vi "Process.vi"(8 "error in":errorcluster, 11 "Oxford1820 UI in":refnum<class "Instrument.OxfordVRM UI.lvclass">) -> (0 "error out":errorcluster, 3 "Oxford1820 UI out":refnum<class "Instrument.OxfordVRM UI.lvclass">)   [LabVIEW 2016, in "Instrument.OxfordVRM UI.lvclass"]
doc: "---------------------------------------------------------------\nJKI State Machine Objects™\nhttp://jki.net/state-machine-objects/\nCopyright (C) 2005-2015, JKI <info@jki.net>\nALL RIGHTS RESERVEDJKI State Machine Objects (SMO) 1.0.0.5\nJKI - JKI\nCopyright (c) 2016, JKI"
uses:
  Instrument.OxfordVRM UI.lvclass
  <vilib>/JKI/JKI SMO/SMO/SMO.lvclass
  <vilib>/JKI/JKI SMO/SMO/Typedefs/Parent Call--Enum.ctl
  <vilib>/JKI/JKI SMO/SMO.UI/SMO.UI.lvclass
  <userlib>/LevyLab/Levylab Instruments/SMOs/Instrument/Instrument.lvclass
  Instrument.Oxford1820/Typedefs/getAll.ctl
  Instrument.Oxford1820/Instrument.OxfordVRM.lvclass
  <userlib>/LevyLab/Levylab Instruments/SMOs/Instrument UI/Instrument UI.lvclass
  Instrument.Oxford1820/Typedefs/Fill Mode-Combo.ctl
  <instrlib>/Mercury iXX/Public/Libraries/Magnet/Controls/Switch Heater.ctl
  <instrlib>/Mercury iXX/Public/Libraries/Magnet.lvlib
  C:/Program Files (x86)/National Instruments/LabVIEW 2016/user.lib/LevyLab/Levylab Instruments/SMOs/Instrument UI/Instrument UI.lvclass
  C:/Program Files (x86)/National Instruments/LabVIEW 2016/vi.lib/JKI/JKI SMO/SMO.UI/SMO.UI.lvclass
  C:/Program Files (x86)/National Instruments/LabVIEW 2016/vi.lib/JKI/JKI SMO/SMO/SMO.lvclass
  C:/Program Files (x86)/National Instruments/LabVIEW 2016/user.lib/LevyLab/Levylab Instruments/Instrument Types/Cryostat/Instrument.Cryostat.lvclass
  C:/Program Files (x86)/National Instruments/LabVIEW 2016/user.lib/LevyLab/Levylab Instruments/SMOs/Instrument/Instrument.lvclass
panel:
  in  "Open Target":dbl=100.0 format="%.1f (%%)"
  out "System Time (HH:MM:SS)":dbl=165.3592643737793 format="%<%I:%M:%S %p>T"
  out "LPF on":dbl format="%<%H:%M:%S>t"
  out "PS Heat on (HH:MM:SS)":dbl format="%<%H:%M:%S>t"
  out "ETA":dbl=3660699600.0 format="%<%I:%M:%S %p %m/%d/%Y>T"
  out "version":string="v20/10/28"
  out "Waveform Chart 2":T1(graph)
  out "N2 LEVEL":dbl format="%.0f %"
  in  "Window Maximize":bool
  in  "Window Minimize":bool
  out "Magnet Status 3":string="Status: Clamped"
  in  "Remote Mode":bool
  out "Sentinel":bool=TRUE
  out "Voltage Meter":dbl(knob) caption="Voltage (V)" scale=-10.0..10.0
  out "Current Meter":dbl(knob) caption="Voltage (V)" scale=-180.0..180.0
  out "Magnet Field Meter":dbl(knob) caption="Voltage (V)" scale=-20.0..20.0
  in  "Hold":bool
  in  "To Set":bool
  in  "Export":bool
  out "PSU Field":dbl format="%#.5f T"
  in  "Target Field (T)":dbl caption="Field" format="%.2f"
  out "Target Field (T)":dbl caption="Field" format="%.2f T"
  in  "Target Rate (T/min)":dbl=0.1 caption="Rate" min=0.0 max=1.0 format="%.2f"
  out "Target Rate (T/min)":dbl caption="Rate" format="%.2f T/min"
  out "Field":dbl format="%.5f T"
  out "He LEVEL":dbl format="%.0f %"
  in  "PS Heat":bool
  in  "To Zero":bool
  in  "Clamp":bool
  out "N2 LVL":dbl format="%.1f (%%)"
  out "He LVL Chart":dbl(slide)=52.0833 scale=0.0..100.0
  out "N2 LVL Chart":dbl(slide)=61.3025 scale=0.0..100.0
  out "He LVL":dbl format="%.1f (%%)"
  in  "Fast/Slow Fill":bool
  in  "Open Needle Valve":bool
  in  "Close Needle Valve":bool
  in  "LPF Power":bool
  out "Needle Valve":dbl format="%.1f (%%)"
  out "Pressure":dbl format="%_5f mB"
  out "Magnet T":dbl format="%_2f K"
  out "Magnet R":dbl format="%_3f ohms"
  out "Voltage":dbl format="%.5f V"
  out "Current":dbl format="%.5f A"
  out "Magnet Status 2":string="Status: Clamped"
  in  "Power":bool
  # "Obsolete controls?"
  # "Actions"
  # "Targets"
  # "Status"
  # "Slow Rates\nCurrent Range (A)     Field Range (T)  Rate (T/min)\n0       -- 100        0    -- 11.5     0.91\n100     -- 150        11.5 -- 17.2     0.23\n150     -- 155.467    17.2 -- 18       0.11\n155.567 -- 172.471    18   -- 20       0.11\n\nFast Rates\nCurrent Range (A)     Field Range (T)  Rate (T/min)\n0       -- 155.467    0    -- 18       1.0\n155.567 -- 172.471    18   -- 20       0.25"
  # "IPS"
  # "PS Switch"
  # "Level"
  # "Level Graph"
  # "LPF"
  # "Helium"
  # "Nitrogen"
  # "^^^^"
  # "Needle Valve"
  # "Slow Rates\nCurrent Range (A)     Field Range (T)   Rate (T/min)\n0       -- 100        0    -- 11.5      0.91\n100     -- 150        11.5 -- 17.2      0.23\n150     -- 155.467    17.2 -- 18        0.11\n155.567 -- 172.471    18   -- 20        0.11\n\nFast Rates\nCurrent Range (A)     Field Range (T)   Rate (T/min)\n0       -- 155.467    0    -- 18        1.0\n155.567 -- 172.471    18   -- 20        0.25"
  # "SMO UI Template"
  # "For instructions on how to use the JKI State Machine Objects, examples and video tutorials, visit:\nhttp://jki.net/state-machine-objects/\n\nJKI State Machine Objects™\nhttp://jki.net/state-machine-objects/\nCopyright (C) 2005-2015, JKI <info@jki.net>\nALL RIGHTS RESERVED"
  # "Voltage (V)"
  # "Current (A)"
  # "Magnet (T)"
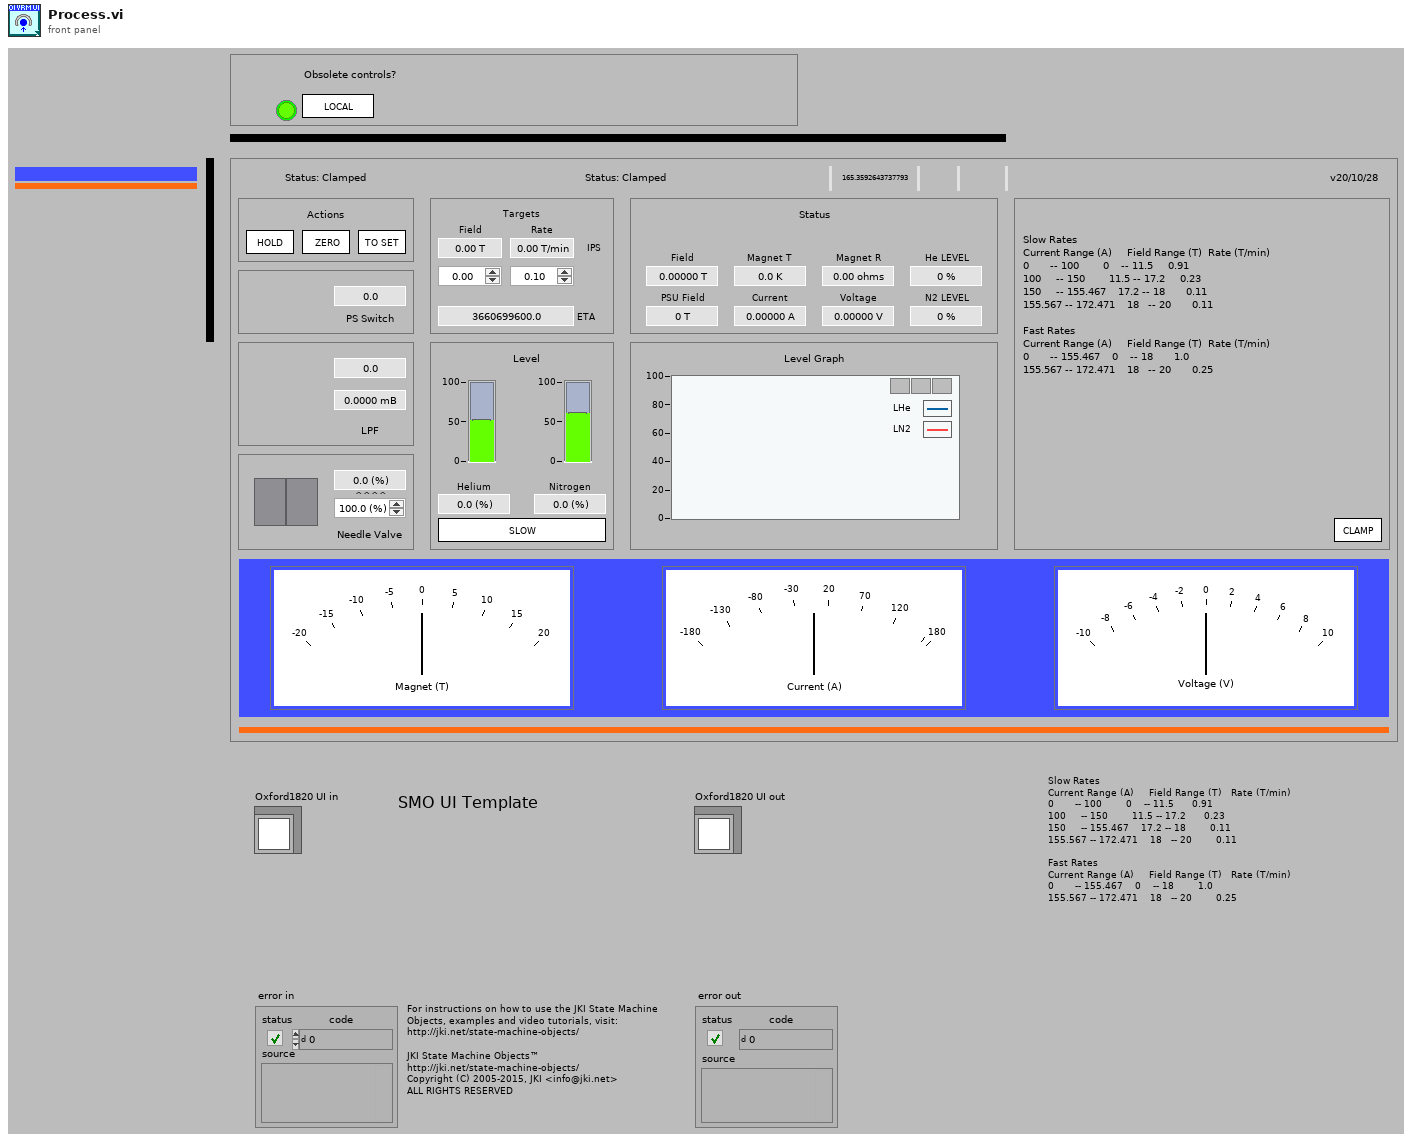
[diagram p1: front panel]
types:
  T1 = cluster{"1820_IPS_Level_He":dbl, "1820_IPS_Level_N2":dbl}
  T2 = typedef "SMO.lvclass/Parent Call--Enum.ctl" = enum16{"Allows parent to run", "Does not request parent to run"}
  T3 = typedef "Mercury iXX.lvlib/Magnet.lvlib/Switch Heater.ctl" = string
  T4 = enum32{"invalid app kind", "Development System", "Run Time System", "Student Edition", "Embedded LabVIEW", "Evaluation", "Custom"}
  T5 = typedef "Instrument.OxfordVRM.lvclass/getAll.ctl" = cluster{"1820_IPS_Magnet_Field":dbl, "1820_IPS_PS_Field":dbl, "1820_IPS_Target_Field":dbl, "1820_IPS_Target_Field_Rate":dbl, "1820_IPS_Voltage":dbl, "1820_IPS_Current":dbl, "1820_IPS_Level_N2":dbl, "1820_IPS_Level_He":dbl, "1820_IPS_Magnet_Temperature":dbl, "1820_IPS_Magnet_Temperature_R":dbl, "1820_IPS_M1_Current":dbl, "1820_IPS_M1_Voltage":dbl, "1820_IPS_M2_Current":dbl, "1820_IPS_M2_Voltage":dbl, "1820_IPS_M3_Current":dbl, "1820_IPS_M3_Voltage":dbl, "1820_IPS_Status":string, "1820_IPS_Switch":string, "1820_ITC_Lambda_Temperature":dbl, "1820_ITC_Lambda_Temperature_R":dbl, "1820_ITC_Pressure":dbl, "1820_ITC_Needle_Valve":dbl}
  T6 = enum32{"Invalid", "Standard", "Closed", "Hidden", "Minimized", "Maximized"}
  T7 = typedef "Instrument.OxfordVRM.lvclass/Fill Mode-Combo.ctl" = string
  T8 = typedef "RemoteControl.lvclass/Message--Cluster.ctl" = cluster{"Command":string, "Data":variant, "Message ID":i32}
  T9 = cluster{"Core":cluster{"Current VI Reference":refnum<vi>, "Close Panel on Exit?":bool, "error":errorcluster}, "Instrument UI out":refnum<class "Instrument.OxfordVRM UI.lvclass">, "Instrument":refnum<class "Instrument.OxfordVRM.lvclass">, "getAll":variant, "Response":string, "config":variant, "switch time":timestamp, "LPF time":timestamp}
  T10 = typedef "Instrument.OxfordVRM.lvclass/PublicEvents--Instrument.Oxford1820.ProcessStatus.ctl" = string
  T11 = cluster{"Current VI Reference":refnum<vi>, "Close Panel on Exit?":bool, "error":errorcluster}
  T12 = typedef "LVRectTypeDef.ctl" = cluster{"Left":i16, "Top":i16, "Right":i16, "Bottom":i16}
  T13 = typedef "SMO.lvclass/Protected Events.ctl" = cluster{"StopProcesses":refnum<user-event>, "AbortProcesses":refnum<user-event>, "Config Changed":refnum<user-event>, "Dependency":refnum<user-event>}
  T14 = typedef "Instrument.lvclass/PublicEvents--Cluster.ctl" = cluster{"MessageFromProcess":refnum<user-event>}
  T15 = typedef "Instrument.OxfordVRM.lvclass/PublicEvents--Cluster.ctl" = cluster{"ProcessStatus":refnum<user-event>}
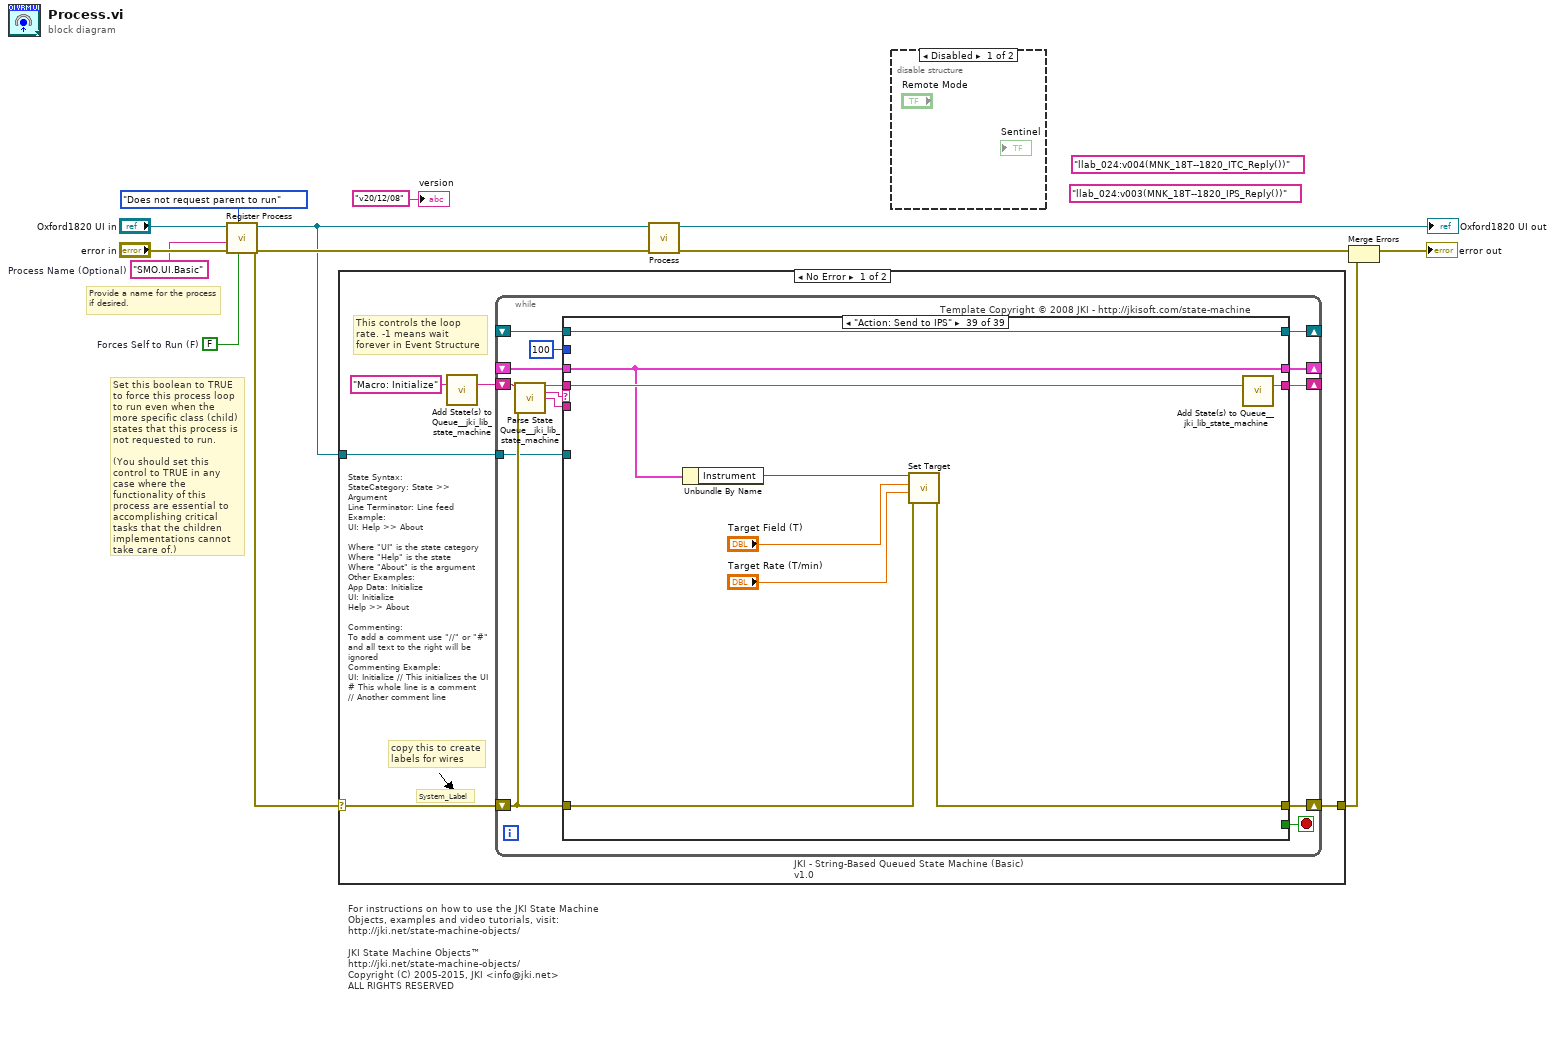
[diagram p0: block diagram]
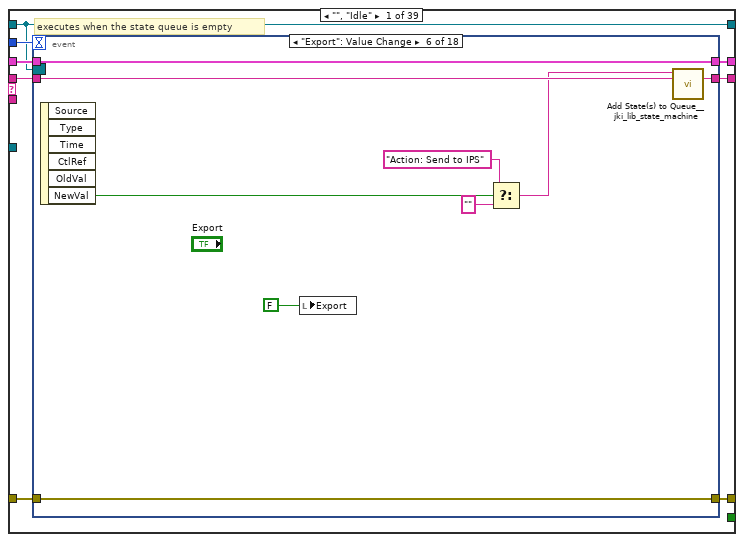
[diagram p3: hidden frame]
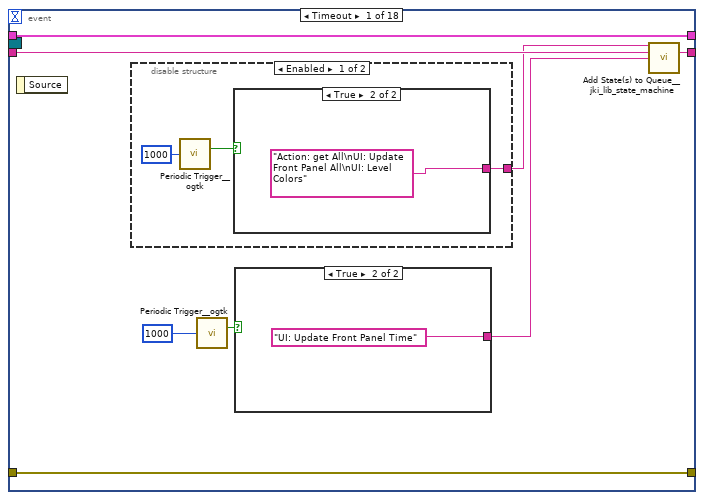
[diagram p4: hidden frame]
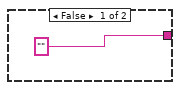
[diagram p5: hidden frame]
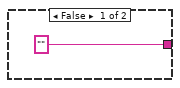
[diagram p6: hidden frame]
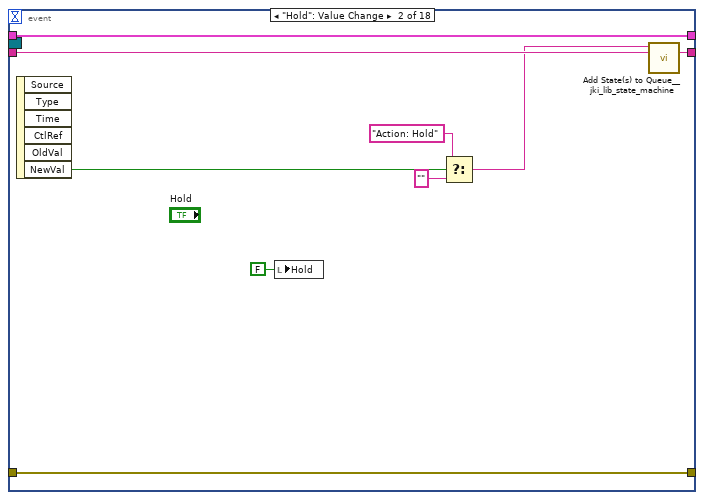
[diagram p8: hidden frame]
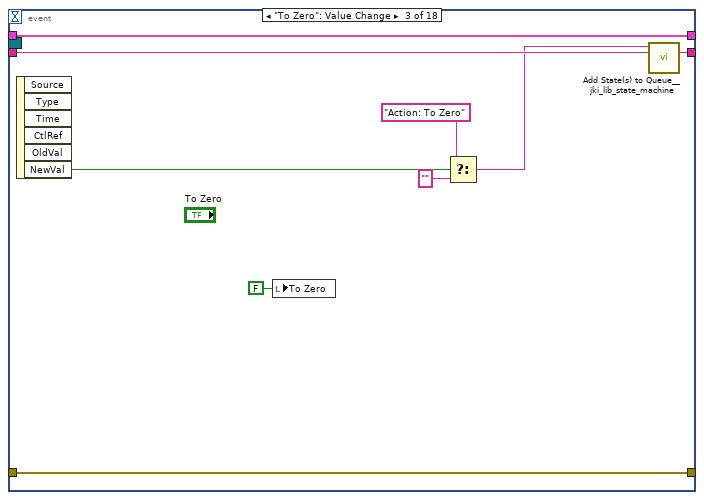
[diagram p9: hidden frame]
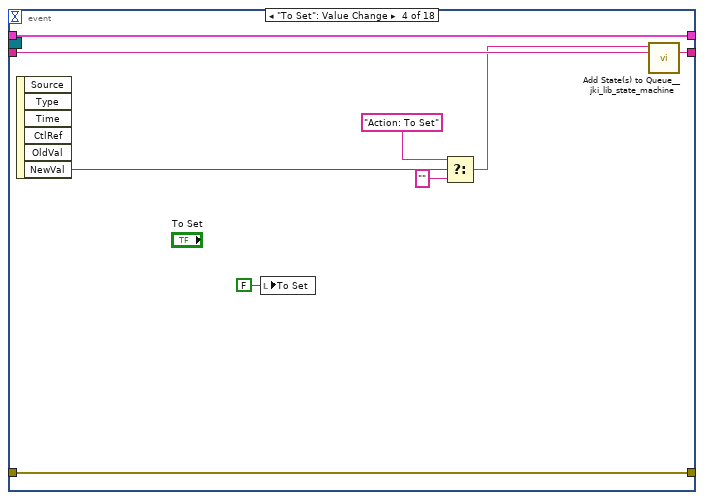
[diagram p10: hidden frame]
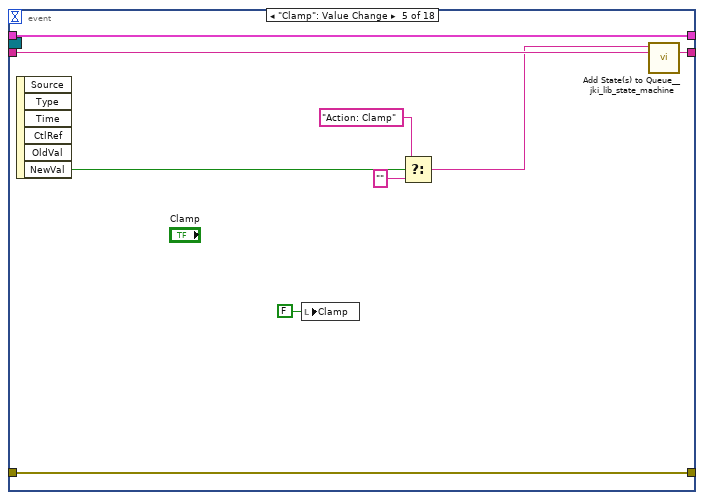
[diagram p11: hidden frame]
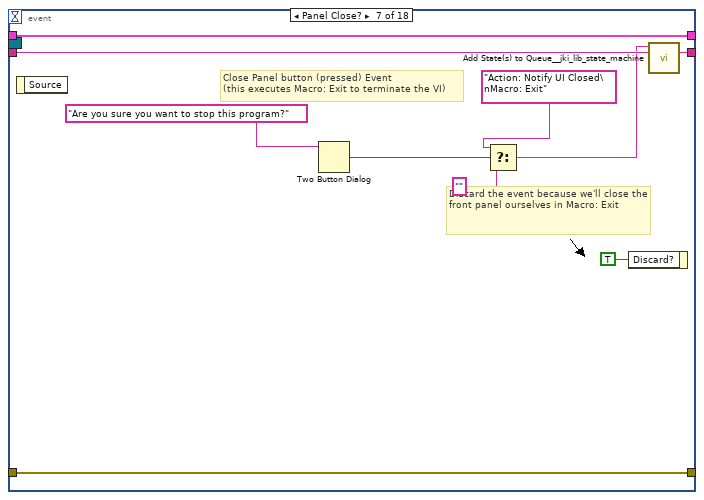
[diagram p12: hidden frame]
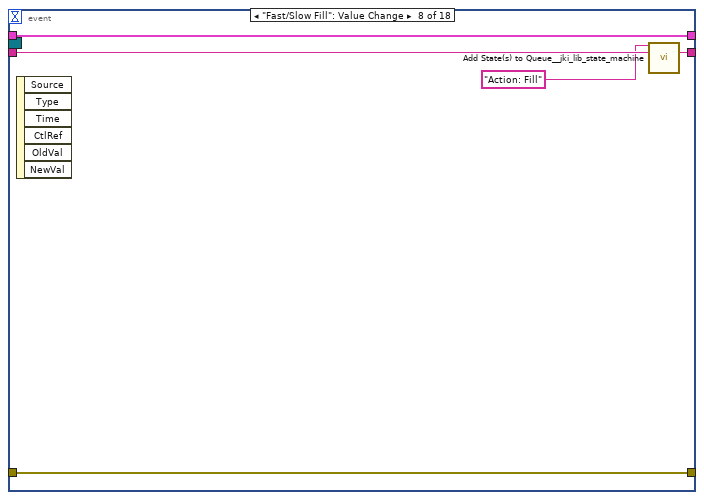
[diagram p13: hidden frame]
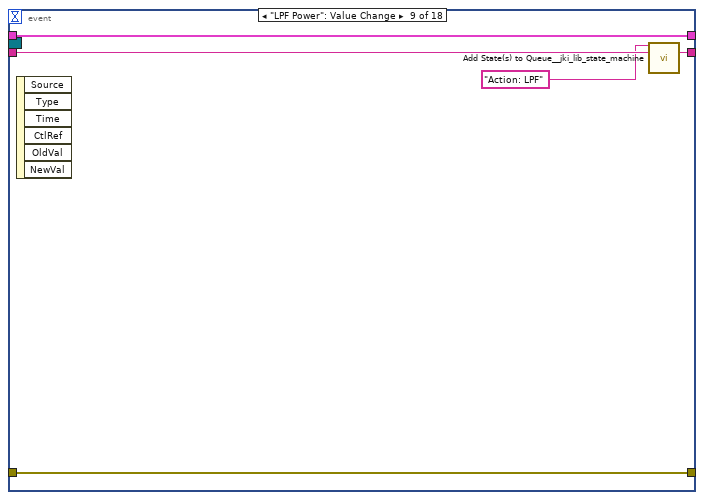
[diagram p14: hidden frame]
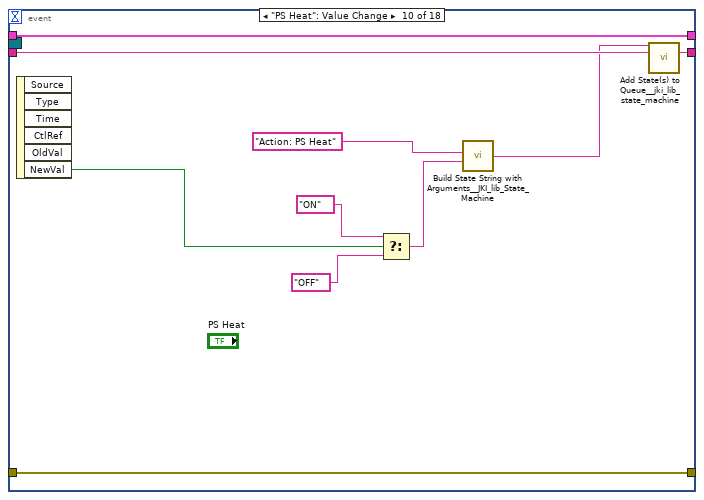
[diagram p15: hidden frame]
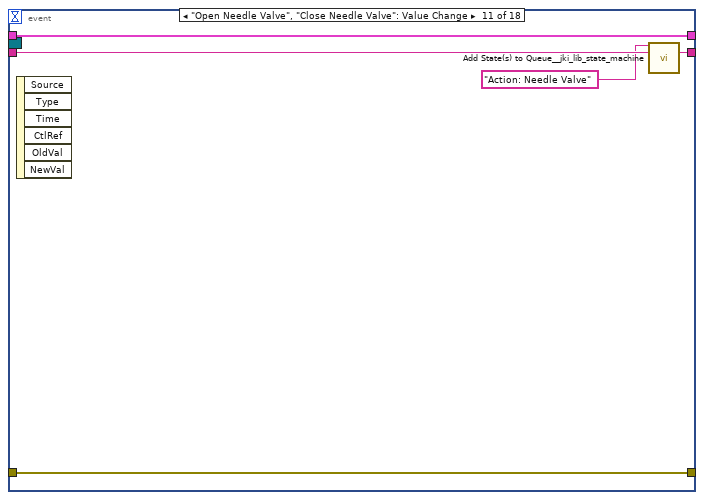
[diagram p16: hidden frame]
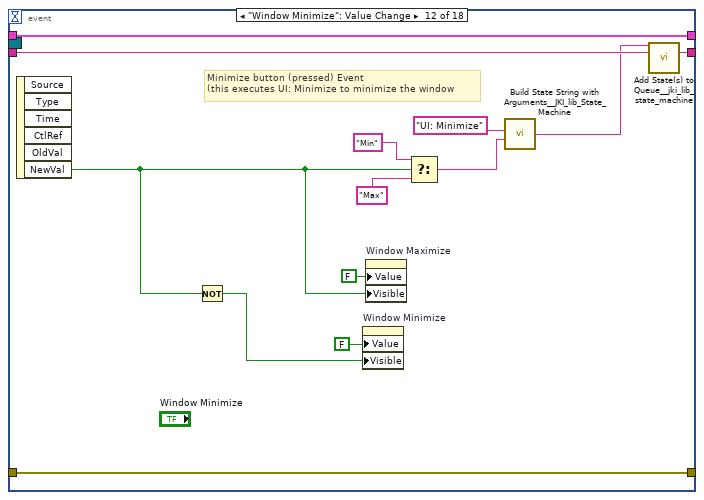
[diagram p17: hidden frame]
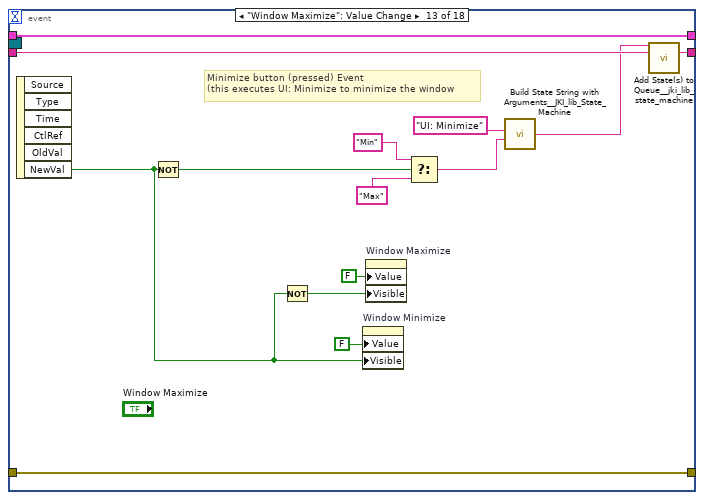
[diagram p18: hidden frame]
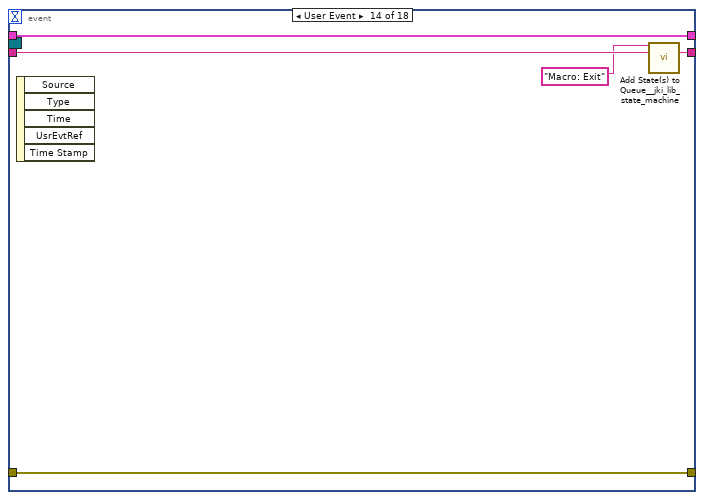
[diagram p19: hidden frame]
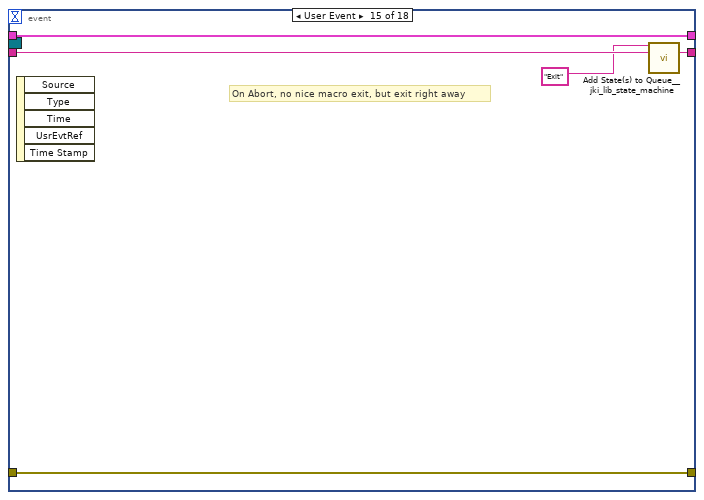
[diagram p20: hidden frame]
diagram:
  (unwired) "llab_024:v004(MNK_18T--1820_ITC_Reply())" ("variable")
  (unwired) "llab_024:v003(MNK_18T--1820_IPS_Reply())" ("variable")
  w3 = FALSE  # Forces Self to Run (F)
  w2 = "SMO.UI.Basic"  # Process Name (Optional)
  # "Provide a name for the process\nif desired."
  # "Set this boolean to TRUE to force this process loop to run even when the more specific class (child) states that this process is not requested to run.\n\n(You should set this control to TRUE in any case where the functionality of this process are essential to accomplishing critical tasks that the children implementations cannot take care of.)"
  # "For instructions on how to use the JKI State Machine Objects, examples and video tutorials, visit:\nhttp://jki.net/state-machine-objects/\n\nJKI State Machine Objects™\nhttp://jki.net/state-machine-objects/\nCopyright (C) 2005-2015, JKI <info@jki.net>\nALL RIGHTS RESERVED"
  n1 = call <vilib>:"Register Process.vi"("Forces Self to Run (F)"=w3, "Parent Call"=Parent_Call--Enum."Does not request parent to run", "error in (no error)"="error in", "Process Name (optional)"=w2, "SMO"="Oxford1820 UI in") -> ("error out"=w9:errorcluster, "SMO out"=w8:refnum<class "Instrument.OxfordVRM UI.lvclass">)  [unwired: 5 in]
  n2 = case shown="No Error" w9 {
    selector: w9 -> [w14 w643]
    tunnel: w8 -> [w15 _]
    tunnel: [w13 w643] -> w5
    frame No Error {
      # "State Syntax:\nStateCategory: State >> Argument\nLine Terminator: Line feed\nExample:\nUI: Help >> About\n\nWhere \"UI\" is the state category\nWhere \"Help\" is the state\nWhere \"About\" is the argument\nOther Examples:\nApp Data: Initialize\nUI: Initialize\nHelp >> About\n\nCommenting:\nTo add a comment use \"//\" or \"#\" and all text to the right will be ignored\nCommenting Example:\nUI: Initialize // This initializes the UI\n# This whole line is a comment\n// Another comment line"
      # "copy this to create labels for wires"
      # "This controls the loop rate. -1 means wait forever in Event Structure"
      # "System_Label"
      n3 = call <vilib>:"Add State(s) to Queue__jki_lib_state_machine.vi"("State(s) in (\"\")"="Macro: Initialize") -> ("States Out"=w17:string)  [unwired: 14 in]
      n4 = while "JKI - String-Based Queued State Machine (Basic) v1.0" {
        shift-right: [w24] -> _
        shift-left: _ -> [w23]
        shift-right: [w27] -> w13
        shift-left: w14 -> [w21]
        shift-right: [w26] -> _
        shift-left: w17 -> [w28]
        tunnel: w15 -> [w20]
        shift-right: [w19] -> _
        shift-left: _ -> [w18]
        stop <- w25 stop-if-true
        # "Template Copyright © 2008 JKI - http://jkisoft.com/state-machine"
        n5 = call <vilib>:"Parse State Queue__jki_lib_state_machine.vi"("State Queue"=w28, "Error In (no error)"=w21) -> ("Remaining States"=w30:string, "Current State"=w31:string, "Arguments"=w29:string)  [unwired: 11 in]
        n6 = case shown="\"Action: Send to IPS\"" w31 {
          selector: w31 -> [_ _ w219 _ _ _ _ _ _ _ _ _ _ _ _ _ _ _ _ _ _ _ _ _ _ _ _ _ _ _ _ _ _ _ _ _ _ _ _]
          tunnel: w30 -> [w39 w217 w223 w242 w256 w262 w267 w290 w297 w302 w313 w339 w358 w364 w371 w378 w394 w428 w454 w463 w477 w482 w493 w500 w505 w521 w527 w534 w541 w551 w560 w567 w574 w581 w592 w605 w618 w633 w642]
          tunnel: w29 -> [_ _ _ _ _ _ _ _ _ _ _ _ _ w359 _ w372 w388 w429 _ _ _ _ _ _ _ _ _ _ _ _ _ _ _ _ _ _ _ w624 _]
          tunnel: w23 -> [w37 w214 w221 w233 w244 w258 w264 _ w292 w299 w311 w336 w354 w361 w368 w376 w390 w427 w451 w459 w468 w479 w490 w495 w502 w519 w525 w530 w537 w542 w557 w564 w571 w575 w589 w595 w615 w628 w639]
          tunnel: [w36 w215 w225 w239 w249 w257 w265 w278 w293 w300 w308 w334 w356 w362 w369 w373 w391 w422 w452 w461 w475 w480 w484 w496 w503 w515 w522 w531 w535 w545 w556 w561 w568 w576 w586 w600 w606 w629 w636] -> w27
          tunnel: w21 -> [w35 w215 w224 w239 w245 _ w265 w287 w294 w300 w309 w335 w356 w362 w369 w374 w392 w423 w452 w461 w475 w480 w485 w497 w503 w510 w523 w531 w536 w546 w553 w562 w569 w577 w587 w601 w613 w630 w637]
          tunnel: [w38 w216 w222 w241 w255 w261 w266 w289 w296 w301 w312 w338 w357 w363 w370 w377 w393 w433 w453 w462 w476 w481 w492 w499 w504 w520 w526 w533 w540 w550 w559 w566 w573 w580 w591 w604 w617 w632 w641] -> w26
          tunnel: [_ _ _ _ _ TRUE _ _ _ _ _ _ _ _ _ _ _ _ _ _ _ _ _ _ _ _ _ _ _ _ _ _ _ _ _ _ _ _ _] -> w25
          tunnel: [w34 w214 w221 w240 w247 w258 w264 w288 w292 w299 w311 w336 w354 w361 w368 w376 w390 w427 w451 w459 w468 w479 w490 w495 w502 w519 w525 w529 w537 w548 w557 w564 w571 w575 w589 w594 w615 w626 w639] -> w24
          tunnel: 100 ("Timeout") -> [w33 _ _ _ _ _ _ _ _ _ _ _ _ _ _ _ _ _ _ _ _ _ _ _ _ _ _ _ _ _ _ _ _ _ _ _ _ _ _]
          tunnel: w20 -> [_ _ _ _ _ _ _ w275 _ _ _ _ _ _ _ _ _ _ _ _ _ _ _ _ _ _ _ _ _ _ _ _ _ _ _ _ _ _ _]
          tunnel: [w32 w213 w218 w230 w254 w259 w263 w285 w291 w298 w310 w337 w355 w360 w367 w375 w387 w432 w450 w460 w469 w478 w491 w498 w501 w518 w524 w532 w539 w549 w558 w565 w572 w579 w590 w603 w616 w631 w640] -> w19
          tunnel: w18 -> [w32 w213 w218 w230 w254 w259 w263 w285 w291 w298 w310 w337 w355 w360 w367 w375 w387 w432 w450 w460 w469 w478 w491 w498 w501 _ w524 w532 w539 w549 w558 w565 w572 w579 w590 w603 w616 w631 w640]
          frame "", "Idle" {
            # "executes when the state queue is empty"
            n7 = event shown="[5] \"Export\": Value Change" {
              selector: w32 -> [_ _ _ _ _ _ _ _ _ _ _ _ _ _ _ _ _ _]
              dyn-events: _ -> [_ _ _ _ _ _ _ _ _ _ _ _ _ _ _ _ _ _]
              timeout: w33 -> [_ _ _ _ _ _ _ _ _ _ _ _ _ _ _ _ _ _]
              tunnel: w39 -> [w47 w63 w72 w81 w90 w99 w109 w114 w119 w129 w134 w147 w161 w166 w171 w180 w190 w212]
              tunnel: [w46 w62 w71 w80 w89 w98 w108 w113 w118 w128 w133 w146 w160 w165 w170 w179 w189 w211] -> w38
              tunnel: w37 -> [w43 w60 w69 w78 w87 w96 w106 w112 w117 w127 w132 w145 w159 w163 w168 w177 w188 w205]
              tunnel: [w45 w61 w70 w79 w88 w97 w105 w111 w116 w126 w131 w144 w158 w164 w169 w178 w181 w209] -> w36
              tunnel: w35 -> [w45 w61 w70 w79 w88 w97 w105 w111 w116 w126 w131 w144 w158 w164 w169 w178 w182 w206]
              tunnel: [w43 w60 w69 w78 w87 w96 w106 w112 w117 w127 w132 w145 w159 w163 w168 w177 w187 w205] -> w34
              event Timeout {
                n8 = event-data() -> ()  [unwired: 1 in, 1 out]
                n9 = disable-structure shown="Enabled" {
                  disable-tunnel: [w50 _] -> w44
                  frame Enabled {
                    n10 = call <userlib>:"Periodic Trigger__ogtk.vi"("time (ms)"=u32 1000 ("update time (ms)")) -> ("Triggered"=w52:bool)  [unwired: 12 in, 2 out]
                    n11 = case shown="True" w52 {
                      tunnel: ["" "Action: get All\nUI: Update Front Panel All\nUI: Level Colors"] -> w50
                      frame False {
                      }
                      frame True {
                      }
                    }
                  }
                  frame Disabled {
                  }
                }
                n12 = call <userlib>:"Periodic Trigger__ogtk.vi"("time (ms)"=u32 1000 ("update time (ms)")) -> ("Triggered"=w41:bool)  [unwired: 12 in, 2 out]
                n13 = case shown="True" w41 {
                  tunnel: ["" "UI: Update Front Panel Time"] -> w40
                  frame False {
                  }
                  frame True {
                  }
                }
                n14 = call <vilib>:"Add State(s) to Queue__jki_lib_state_machine.vi"("State(s) in Front (\"\")"=w44, "State(s) in (\"\")"=w47, "State(s) at Back (\"\")"=w40) -> ("States Out"=w46:string)  [unwired: 12 in]
              }
              event "Hold": Value Change {
                n15 = event-data() -> ("NewVal"=w59:bool)  [unwired: 1 in, 5 out]
                n16 = local write "Hold"(FALSE ("Hold")) -> ()
                n17 = Select(t="Action: Hold" ("State(s) in Front (\"\")"), s=w59, f="") -> (s? t:f=w56:string)
                n18 = call <vilib>:"Add State(s) to Queue__jki_lib_state_machine.vi"("State(s) in Front (\"\")"=w56, "State(s) in (\"\")"=w63) -> ("States Out"=w62:string)  [unwired: 13 in]
              }
              event "To Zero": Value Change {
                n19 = event-data() -> ("NewVal"=w67:bool)  [unwired: 1 in, 5 out]
                n20 = local write "To Zero"(FALSE ("To Zero")) -> ()
                n21 = Select(t="Action: To Zero" ("State(s) in Front (\"\")"), s=w67, f="") -> (s? t:f=w65:string)
                n22 = call <vilib>:"Add State(s) to Queue__jki_lib_state_machine.vi"("State(s) in Front (\"\")"=w65, "State(s) in (\"\")"=w72) -> ("States Out"=w71:string)  [unwired: 13 in]
              }
              event "To Set": Value Change {
                n23 = event-data() -> ("NewVal"=w76:bool)  [unwired: 1 in, 5 out]
                n24 = local write "To Set"(FALSE ("To Set")) -> ()
                n25 = Select(t="Action: To Set" ("State(s) in Front (\"\")"), s=w76, f="") -> (s? t:f=w74:string)
                n26 = call <vilib>:"Add State(s) to Queue__jki_lib_state_machine.vi"("State(s) in Front (\"\")"=w74, "State(s) in (\"\")"=w81) -> ("States Out"=w80:string)  [unwired: 13 in]
              }
              event "Clamp": Value Change {
                n27 = event-data() -> ("NewVal"=w85:bool)  [unwired: 1 in, 5 out]
                n28 = local write "Clamp"(FALSE ("Clamp")) -> ()
                n29 = Select(t="Action: Clamp" ("State(s) in Front (\"\")"), s=w85, f="") -> (s? t:f=w83:string)
                n30 = call <vilib>:"Add State(s) to Queue__jki_lib_state_machine.vi"("State(s) in Front (\"\")"=w83, "State(s) in (\"\")"=w90) -> ("States Out"=w89:string)  [unwired: 13 in]
              }
              event "Export": Value Change {
                n31 = event-data() -> ("NewVal"=w95:bool)  [unwired: 1 in, 5 out]
                n32 = local write "Export"(FALSE ("Send to IPS")) -> ()
                n33 = Select(t="Action: Send to IPS" ("State(s) in Front (\"\")"), s=w95, f="") -> (s? t:f=w92:string)
                n34 = call <vilib>:"Add State(s) to Queue__jki_lib_state_machine.vi"("State(s) in Front (\"\")"=w92, "State(s) in (\"\")"=w99) -> ("States Out"=w98:string)  [unwired: 13 in]
              }
              event Panel Close? {
                # "Discard the event because we'll close the front panel ourselves in Macro: Exit"
                # "Close Panel button (pressed) Event\n(this executes Macro: Exit to terminate the VI)"
                n35 = event-data() -> ()  [unwired: 1 in, 1 out]
                n36 = Two Button Dialog(message="Are you sure you want to stop this program?") -> (T button?=w104:bool)  [unwired: 2 in]
                n37 = Select(t="Action: Notify UI Closed\nMacro: Exit", s=w104, f="") -> (s? t:f=w100:string)
                n38 = event-data("Discard?"=TRUE) -> ()  [unwired: 1 in, 1 out]
                n39 = call <vilib>:"Add State(s) to Queue__jki_lib_state_machine.vi"("State(s) in Front (\"\")"=w100, "State(s) in (\"\")"=w109) -> ("States Out"=w108:string)  [unwired: 13 in]
              }
              event "Fast/Slow Fill": Value Change {
                n40 = event-data() -> ()  [unwired: 1 in, 6 out]
                n41 = call <vilib>:"Add State(s) to Queue__jki_lib_state_machine.vi"("State(s) in Front (\"\")"="Action: Fill", "State(s) in (\"\")"=w114) -> ("States Out"=w113:string)  [unwired: 13 in]
              }
              event "LPF Power": Value Change {
                n42 = event-data() -> ()  [unwired: 1 in, 6 out]
                n43 = call <vilib>:"Add State(s) to Queue__jki_lib_state_machine.vi"("State(s) in Front (\"\")"="Action: LPF", "State(s) in (\"\")"=w119) -> ("States Out"=w118:string)  [unwired: 13 in]
              }
              event "PS Heat": Value Change {
                n44 = event-data() -> ("NewVal"=w120:bool)  [unwired: 1 in, 5 out]
                n45 = Select(t=T3 "ON" ("LPF State"), s=w120, f=T3 "OFF" ("LPF State")) -> (s? t:f=w122:T3)
                n46 = call <vilib>:"Build State String with Arguments__JKI_lib_State_Machine.vi"("Arguments (\"\")"=w122, "State"="Action: PS Heat") -> ("State with Arguments"=w121:string)  [unwired: 4 in]
                n47 = call <vilib>:"Add State(s) to Queue__jki_lib_state_machine.vi"("State(s) in Front (\"\")"=w121, "State(s) in (\"\")"=w129) -> ("States Out"=w128:string)  [unwired: 13 in]
              }
              event "Open Needle Valve", "Close Needle Valve": Value Change {
                n48 = event-data() -> ()  [unwired: 1 in, 6 out]
                n49 = call <vilib>:"Add State(s) to Queue__jki_lib_state_machine.vi"("State(s) in Front (\"\")"="Action: Needle Valve", "State(s) in (\"\")"=w134) -> ("States Out"=w133:string)  [unwired: 13 in]
              }
              event "Window Minimize": Value Change {
                # "Minimize button (pressed) Event\n(this executes UI: Minimize to minimize the window"
                n50 = event-data() -> ("NewVal"=w135:bool)  [unwired: 1 in, 5 out]
                n51 = Not(x=w135) -> (.not. x?=w136:bool)
                n52 = property on="Window Minimize" class="Bool (strict)"("Value"=FALSE ("Window Maximize"), "Visible"=w136) -> ()  [unwired: 2 in, 2 out]
                n53 = property on="Window Maximize" class="Bool (strict)"("Value"=FALSE ("Window Maximize"), "Visible"=w135) -> ()  [unwired: 2 in, 2 out]
                n54 = Select(t="Min" ("Arguments (\"\")"), s=w135, f="Max" ("Arguments (\"\")")) -> (s? t:f=w140:string)
                n55 = call <vilib>:"Build State String with Arguments__JKI_lib_State_Machine.vi"("Arguments (\"\")"=w140, "State"="UI: Minimize") -> ("State with Arguments"=w139:string)  [unwired: 4 in]
                n56 = call <vilib>:"Add State(s) to Queue__jki_lib_state_machine.vi"("State(s) in Front (\"\")"=w139, "State(s) in (\"\")"=w147) -> ("States Out"=w146:string)  [unwired: 13 in]
              }
              event "Window Maximize": Value Change {
                # "Minimize button (pressed) Event\n(this executes UI: Minimize to minimize the window"
                n57 = event-data() -> ("NewVal"=w149:bool)  [unwired: 1 in, 5 out]
                n58 = Not(x=w149) -> (.not. x?=w150:bool)
                n59 = Not(x=w149) -> (.not. x?=w148:bool)
                n60 = property on="Window Minimize" class="Bool (strict)"("Value"=FALSE ("Window Maximize"), "Visible"=w149) -> ()  [unwired: 2 in, 2 out]
                n61 = property on="Window Maximize" class="Bool (strict)"("Value"=FALSE ("Window Maximize"), "Visible"=w148) -> ()  [unwired: 2 in, 2 out]
                n62 = Select(t="Min" ("Arguments (\"\")"), s=w150, f="Max" ("Arguments (\"\")")) -> (s? t:f=w154:string)
                n63 = call <vilib>:"Build State String with Arguments__JKI_lib_State_Machine.vi"("Arguments (\"\")"=w154, "State"="UI: Minimize") -> ("State with Arguments"=w153:string)  [unwired: 4 in]
                n64 = call <vilib>:"Add State(s) to Queue__jki_lib_state_machine.vi"("State(s) in Front (\"\")"=w153, "State(s) in (\"\")"=w161) -> ("States Out"=w160:string)  [unwired: 13 in]
              }
              event User Event {
                n65 = event-data() -> ()  [unwired: 1 in, 5 out]
                n66 = call <vilib>:"Add State(s) to Queue__jki_lib_state_machine.vi"("State(s) in Front (\"\")"="Macro: Exit", "State(s) in (\"\")"=w166) -> ("States Out"=w165:string)  [unwired: 13 in]
              }
              event User Event {
                # "On Abort, no nice macro exit, but exit right away"
                n67 = event-data() -> ()  [unwired: 1 in, 5 out]
                n68 = call <vilib>:"Add State(s) to Queue__jki_lib_state_machine.vi"("State(s) in Front (\"\")"="Exit", "State(s) in (\"\")"=w171) -> ("States Out"=w170:string)  [unwired: 13 in]
              }
              event "Power": Value Change {
                # "if user pushes stop button, give them a window to make sure they\nmeant to stop this program"
                n69 = event-data() -> ()  [unwired: 1 in, 6 out]
                n70 = Two Button Dialog(message="Are you sure you want to stop this program?") -> (T button?=w176:bool)  [unwired: 2 in]
                n71 = Select(t="Macro: Exit", s=w176, f="") -> (s? t:f=w172:string)
                n72 = call <vilib>:"Add State(s) to Queue__jki_lib_state_machine.vi"("State(s) in Front (\"\")"=w172, "State(s) in (\"\")"=w180) -> ("States Out"=w179:string)  [unwired: 13 in]
              }
              event User Event {
                # "#todo: the instrument process will communicate to the UI using Public Events\nFilter the events here to update the UI display, for example"
                n73 = event-data() -> ("Message"=w183:T8)  [unwired: 1 in]
                n74 = Unbundle By Name(w183) -> ("Command"=w185:string, "Data"=w186:variant)
                n75 = case shown="\"getAll\"" w185 {
                  tunnel: w186 -> [w195 w203]
                  tunnel: w188 -> [w194 w204]
                  tunnel: [w193 w204] -> w187
                  tunnel: ["UI: Update Front Panel All" w200] -> w184
                  tunnel: w182 -> [w191 w197]
                  tunnel: [w191 w196] -> w181
                  frame "getAll" {
                    n76 = Bundle By Name(cluster=w194, "getAll"=w195) -> (w193:T9)
                  }
                  frame Default {
                    n77 = Variant To Data(error in=w197, type="", Variant=w203) -> (data=w199:string, error out=w198:errorcluster)
                    n78 = Format Into String(format string="UI: Status 2 >> %s", error in=w198, w199) -> (resulting string=w200:string, error out=w196:errorcluster)  [unwired: 1 in]
                  }
                }
                n79 = call <vilib>:"Add State(s) to Queue__jki_lib_state_machine.vi"("State(s) in Front (\"\")"=w184, "State(s) in (\"\")"=w190) -> ("States Out"=w189:string)  [unwired: 13 in]
              }
              event User Event {
                # "#todo: the instrument process will communicate to the UI using Public Events\nFilter the events here to update the UI display, for example"
                n80 = event-data() -> ("ProcessStatus"=w207:T10)  [unwired: 1 in]
                n81 = Format Into String(format string="UI: Status 2 >> %s", error in=w206, w207) -> (resulting string=w210:string, error out=w209:errorcluster)  [unwired: 1 in]
                n82 = call <vilib>:"Add State(s) to Queue__jki_lib_state_machine.vi"("State(s) in Front (\"\")"=w210, "State(s) in (\"\")"=w212) -> ("States Out"=w211:string)  [unwired: 13 in]
              }
            }
          }
          frame "---------- Core ----------" {
            # "Do not put any code in this frame.\n(it is a separator no-op)"
            n83 = call <vilib>:"Add State(s) to Queue__jki_lib_state_machine.vi"("State(s) in (\"\")"=w217) -> ("States Out"=w216:string)  [unwired: 14 in]
          }
          frame Default {
            w228 = 42 items=["No error", "Argument error", "Memory is full", "Out of zone", "End of file", "File already open", "Generic file I/O error", "File not found", "File permission error", "Disk is full", "Duplicate path", "Too many files open", "System feature not enabled", "Resource file not found", "Cannot add resource", "Resource not found", "Image not found", "Image memory error", "Pen does not exist", "Config type invalid", "Config token not found", "Config parse error", "Config memory error", "Bad external code format", "Bad external code offset", "External code not present", "Null window", "Destroy window error", "Null menu", "Print aborted", "Bad print record", "Print driver error", "Windows error during printing", "Memory error during printing", "Print dialog error", "Generic print error", "Invalid device refnum", "Device not found", "Device parameter error", "Device unit error", "Cannot open device", "Device call aborted", "Generic error", "Cancelled by user", "Object ID too low", "Object ID too high", "Object not in heap", "Unknown heap", "Unknown object (invalid DefProc)", "Unknown object (DefProc not in table)", "Message out of range", "Invalid (null) method", "Unknown message", "Manager call not supported", "Bad address", "Network operation in progress", "Network operation timed out", "Connection is busy", "Network attribute not supported", "Network error", "Address in use", "System out of memory", "Connection aborted", "Connection refused", "Not connected", "Already connected", "Connection closed", "Initialization error (interapplication manager)", "Bad occurrence", "Wait on unbound occurrence handler", "Occurrence queue overflow", "Datalog type conflict", "Unused", "Unrecognized type (interapplication manager)", "Memory corrupt", "Failed to make temporary DLL", "Old CIN version", "Drag socket not found", "Failed to load drop-object", "Failed to register OLE object", "Failed to release OLE object", "Format specifier type mismatch", "Unknown format specifier", "Too few format specifiers", "Too many format specifiers", "Scan failed", "Newer CIN version", "Error converting to variant", "Runtime menu error", "Password tampered", "Variant attribute not found", "Incompatible variant data type", "Event data is not available", "Event Store is not present", "Occurrence is not found", "Event Queue is not created", "Event info is not available", "Refnum passed is NULL", "Error retrieving Class GUID", "Error retrieving CoClass GUID", "Error retrieving TypeLib GUID.", "Bad built application magic bytes.", "Specific driver is different from the specific driver associated with the Logical Name.", "There is no session opened to the class driver.", "Max Error", "MAX - Error with config objects", "MAX - Error loading configuration", "MAX - Group not supported"]
            # "Current State"
            # "Do not delete, rename, or modify this frame.\n(this is used to capture unhandled states and typos)"
            # "Handle mistyped state name (developer tool)"
            n84 = Format Into String(format string="Software Exception: Unhandled State \"%s\"." ("message"), error in=w224, w219) -> (resulting string=w227:string, error out=w226:errorcluster)  [unwired: 1 in]
            n85 = call <vilib>:"Error Cluster From Error Code.vi"("show call chain? (False)"=TRUE, "error in (no error)"=w226, "error message (\"\")"=w227, "error code (0)"=w228) -> ("error out"=w225:errorcluster)  [unwired: 5 in]
            n86 = call <vilib>:"Add State(s) to Queue__jki_lib_state_machine.vi"("State(s) in (\"\")"=w223) -> ("States Out"=w222:string)  [unwired: 14 in]
          }
          frame "Initialize Core Data" {
            # "Do not delete, rename, or modify this frame.\n(this is used to determine panel behavior on exit)"
            # "originally closed?"
            # "exe?"
            # "If panel starts closed or is an EXE, then close it when we exit"
            n87 = property class="VI"() -> ("Front Panel.Open"=w238:bool)  [unwired: 2 in, 2 out]
            n88 = property class="App"() -> ("App.Kind"=w237:T4)  [unwired: 2 in, 2 out]
            n89 = control-ref of="Current VI Reference"() -> (w231:refnum<vi>)
            n90 = Not(x=w238) -> (.not. x?=w235:bool)
            n91 = Equal?(x=w237, y=T4."Run Time System" ("Application:Kind")) -> (x = y?=w234:bool)
            n92 = Or(x=w235, y=w234) -> (x .or. y?=w232:bool)
            n93 = Bundle By Name(cluster=w233, "Core.Current VI Reference"=w231, "Core.Close Panel on Exit?"=w232) -> (w240:T9)
            n94 = call <vilib>:"Add State(s) to Queue__jki_lib_state_machine.vi"("State(s) in (\"\")"=w242) -> ("States Out"=w241:string)  [unwired: 14 in]
          }
          frame "Error Handler" {
            w249 = errorcluster {"status"=FALSE, "code"=0, "source"=""}  # No error
            # "Overwrite this method to handle errors and pass to parent if not handled. Parent will fire a public event if the error is not handled up the chain of classes."
            # "Handle any errors here.\nYou can also output any states to clean-up after errors occur"
            n95 = Unbundle By Name(w244) -> ("Instrument UI out"=w253:refnum<class "Instrument.OxfordVRM UI.lvclass">)
            n96 = call-dynamic "Handle Error.vi"("Stop on Unhandled Error (T)"=FALSE, "error in"=w245, "Instrument.Oxford1820 UI"=w253) -> ("handling error"=w243:errorcluster, "Unhandled error"=w248:errorcluster)  [unwired: 6 in, 1 out]
            n97 = Bundle By Name(cluster=w244, "Core.error"=w248) -> (w247:T9)
            n98 = Select(t="Exit", s=w243, f="") -> (s? t:f=w250:string)
            n99 = call <vilib>:"Add State(s) to Queue__jki_lib_state_machine.vi"("State(s) in Front (\"\")"=w250, "State(s) in (\"\")"=w256) -> ("States Out"=w255:string)  [unwired: 13 in]
          }
          frame "Exit" {
            # "Do not put any code in this frame.\n(No errors that occur here will be handled.)"
            n100 = Unbundle By Name(w258) -> ("Core.error"=w257:errorcluster)
            n101 = call <vilib>:"Add State(s) to Queue__jki_lib_state_machine.vi"("State(s) in (\"\")"=w262) -> ("States Out"=w261:string)  [unwired: 14 in]
          }
          frame "---------- Data ----------" {
            # "Do not put any code in this frame.\n(It is a separator no-op. You can make a copy of this frame to create a new Data frame)"
            n102 = call <vilib>:"Add State(s) to Queue__jki_lib_state_machine.vi"("State(s) in (\"\")"=w267) -> ("States Out"=w266:string)  [unwired: 14 in]
          }
          frame "Data: Initialize" {
            w268 = refnum<class "Instrument.OxfordVRM.lvclass"> refnum  # Instrument
            w276 = timestamp(0 s since 1904-01-01)  # LPF time
            w280 = timestamp(0 s since 1904-01-01)  # switch time
            w281 = variant  # config
            w282 = ""  # Response
            w283 = variant  # getAll
            w284 = T11 {"Current VI Reference"=refnum, "Close Panel on Exit?"=FALSE, "error"={"status"=FALSE, "code"=0, "source"=""}}  # Core
            w286 = refnum<class "Instrument.OxfordVRM UI.lvclass"> refnum  # Self Reference
            # "do not delete - used by framework"
            # "Data names and types of shift register data are defined by this bundle."
            # "Initialize the shift-register data, here.\n(data names are defined by what you wire into the bundle function)"
            n103 = Variant To Data(error in=w287, type=w286, Variant=w275) -> (data=w274:refnum<class "Instrument.OxfordVRM UI.lvclass">, error out=w273:errorcluster)
            n104 = call <userlib>:"Read Instrument.vi"("error in (no error)"=w273, "Instrument UI in"=w274) -> ("error out"=w272:errorcluster, "Instrument.lvclass"=w269:refnum<class "Instrument.lvclass">, "Instrument UI out"=w270:refnum<class "Instrument.OxfordVRM UI.lvclass">)  [unwired: 7 in]
            n105 = To More Specific Class(target class=w268, reference=w269) -> (specific class reference=w271:refnum<class "Instrument.OxfordVRM.lvclass">)  [unwired: 1 in, 1 out]
            n106 = Get Date/Time In Seconds() -> (seconds since 1Jan1904=w279:timestamp)
            n107 = Variant To Data(error in=w272, type=w280, Variant=w279) -> (data=w277:timestamp, error out=w278:errorcluster)
            n108 = Bundle("Core"=w284, "Instrument UI out"=w270, "Instrument"=w271, "getAll"=w283, "Response"=w282, "config"=w281, "switch time"=w277, "LPF time"=w276) -> (w288:T9)  [unwired: 1 in]
            n109 = call <vilib>:"Add State(s) to Queue__jki_lib_state_machine.vi"("State(s) in (\"\")"=w290) -> ("States Out"=w289:string)  [unwired: 14 in]
          }
          frame "Data: Cleanup" {
            # "Cleanup any data and references, here.\n(this is called automatically, by the Macro: Exit)"
            n110 = Unbundle By Name(w292) -> ("Core.Current VI Reference"=w295:refnum<vi>)
            n111 = Close Reference(reference=w295, error in (no error)=w294) -> (error out=w293:errorcluster)
            n112 = call <vilib>:"Add State(s) to Queue__jki_lib_state_machine.vi"("State(s) in (\"\")"=w297) -> ("States Out"=w296:string)  [unwired: 14 in]
          }
          frame "---------- UI ----------" {
            # "Do not put any code in this frame.\n(It is a separator no-op. You can make a copy of this frame to create a new UI frame)"
            n113 = call <vilib>:"Add State(s) to Queue__jki_lib_state_machine.vi"("State(s) in (\"\")"=w302) -> ("States Out"=w301:string)  [unwired: 14 in]
          }
          frame "UI: Initialize" {
            # "size window to decoration box on front panel"
            # "Initialize the User Interface, here.\n(this is called automatically, by the Macro: Init)"
            n114 = property on="Window Minimize" class="Bool (strict)"("Value"=FALSE ("Window Maximize"), "Visible"=TRUE ("Window Maximize")) -> ()  [unwired: 2 in, 2 out]
            n115 = property on="Window Maximize" class="Bool (strict)"("Value"=FALSE ("Window Maximize"), "Visible"=FALSE ("Window Maximize")) -> ()  [unwired: 2 in, 2 out]
            n116 = invoke on="Power" class="Bool (strict)" method="Reinit To Default"() -> ()  [unwired: 3 in, 3 out]
            n117 = call <userlib>:"Fit VI window to Largest Dec__ogtk.vi"("error in (no error)"=w309, "border spacing (2 px)"=0) -> ("error out"=w308:errorcluster)  [unwired: 4 in, 1 out]
            n118 = call <vilib>:"Add State(s) to Queue__jki_lib_state_machine.vi"("State(s) in (\"\")"=w313) -> ("States Out"=w312:string)  [unwired: 14 in]
          }
          frame "UI: Update Front Panel All" {
            n119 = Unbundle By Name(w336) -> ("getAll"=w333:variant)
            n120 = Variant To Data(error in=w335, type=T5 {"1820_IPS_Magnet_Field"=0.0, "1820_IPS_PS_Field"=0.0, "1820_IPS_Target_Field"=0.0, "1820_IPS_Target_Field_Rate"=0.0, "1820_IPS_Voltage"=0.0, "1820_IPS_Current"=0.0, "1820_IPS_Level_N2"=0.0, "1820_IPS_Level_He"=0.0, "1820_IPS_Magnet_Temperature"=0.0, "1820_IPS_Magnet_Temperature_R"=0.0, "1820_IPS_M1_Current"=0.0, "1820_IPS_M1_Voltage"=0.0, "1820_IPS_M2_Current"=0.0, "1820_IPS_M2_Voltage"=0.0, "1820_IPS_M3_Current"=0.0, "1820_IPS_M3_Voltage"=0.0, "1820_IPS_Status"="", "1820_IPS_Switch"="", "1820_ITC_Lambda_Temperature"=0.0, "1820_ITC_Lambda_Temperature_R"=0.0, "1820_ITC_Pressure"=0.0, "1820_ITC_Needle_Valve"=0.0} ("getAll"), Variant=w333) -> (data=w331:T5, error out=w334:errorcluster)
            n121 = Unbundle By Name(w331) -> ("1820_IPS_Magnet_Field"=→"Field" →"Magnet Field Meter":dbl, "1820_IPS_PS_Field"=→"PSU Field":dbl, "1820_IPS_Target_Field"=→"Target Field (T)":dbl, "1820_IPS_Target_Field_Rate"=→"Target Rate (T/min)":dbl, "1820_IPS_Voltage"=→"Voltage" →"Voltage Meter":dbl, "1820_IPS_Current"=→"Current" →"Current Meter":dbl, "1820_IPS_Level_N2"=w316:dbl, "1820_IPS_Level_He"=w317:dbl, "1820_IPS_Status"=w318:string, "1820_IPS_Switch"=w315:string, "1820_ITC_Lambda_Temperature"=→"Magnet T":dbl, "1820_ITC_Lambda_Temperature_R"=→"Magnet R":dbl, "1820_ITC_Pressure"=→"Pressure":dbl, "1820_ITC_Needle_Valve"=→"Needle Valve":dbl)  [unwired: 8 out]
            "He LEVEL" <- w317
            "He LVL" <- w317
            "He LVL Chart" <- w317
            "N2 LVL Chart" <- w316
            "N2 LVL" <- w316
            "N2 LEVEL" <- w316
            n122 = call "Switch Status String to Boolean.vi"("String"=w315) -> ("Switch:"=w314:bool)
            n123 = call "Action Status to Text.vi"("PSU Act Stat"=w318) -> ("Status:"=→"Magnet Status 3":string)
            n124 = local write "PS Heat"(w314) -> ()
            n125 = Bundle("1820_IPS_Level_He"=w317, "1820_IPS_Level_N2"=w316) -> (→"Waveform Chart 2":T1)  [unwired: 1 in]
            n126 = call <vilib>:"Add State(s) to Queue__jki_lib_state_machine.vi"("State(s) in (\"\")"=w339) -> ("States Out"=w338:string)  [unwired: 14 in]
          }
          frame "UI: Update Front Panel Time" {
            # "Do not put any code in this frame.\n(It is a separator no-op. You can make a copy of this frame to create a new UI frame)"
            n127 = Unbundle By Name(w354) -> ("switch time"=w352:timestamp, "LPF time"=w351:timestamp)
            n128 = Get Date/Time In Seconds() -> (seconds since 1Jan1904=w344:timestamp)
            n129 = local read "LPF Power"() -> (w348:bool)
            n130 = local read "PS Heat"() -> (w340:bool)
            n131 = local read "Target Rate (T/min)"() -> (w346:dbl)
            n132 = local read "Target Field (T)"() -> (w349:dbl)
            n133 = local read "PSU Field"() -> (w345:dbl)
            n134 = local read "Field"() -> (w347:dbl)
            n135 = To Double Precision Float(number=w344) -> (double precision float=→"System Time (HH:MM:SS)":dbl)
            n136 = call "1820 PS Heat duration.vi"("PS Heat"=w340, "time stamp"=w352) -> ("PS Heat on (HH:MM:SS)"=→"PS Heat on (HH:MM:SS)":dbl)  [unwired: 9 in]
            n137 = call "1820 LPF ON duration.vi"("Lambda"=w348, "LPF ON"=w351) -> ("LPF on (HH:MM:SS)"=→"LPF on":dbl)  [unwired: 9 in]
            n138 = call "1820 Sweep ETA.vi"("Power Supply Field (T)"=w345, "Target Field Rate (T/min)"=w346, "Magnet Field (T)"=w347, "Target Field (T)"=w349) -> ("ETA timestamp"=w342:timestamp)  [unwired: 5 in, 2 out]
            n139 = To Double Precision Float(number=w342) -> (double precision float=→"ETA":dbl)
            n140 = call <vilib>:"Add State(s) to Queue__jki_lib_state_machine.vi"("State(s) in (\"\")"=w358) -> ("States Out"=w357:string)  [unwired: 14 in]
          }
          frame "UI: Status 2" {
            # "Do not put any code in this frame.\n(It is a separator no-op. You can make a copy of this frame to create a new UI frame)"
            n141 = call <vilib>:"Add State(s) to Queue__jki_lib_state_machine.vi"("State(s) in (\"\")"=w364) -> ("States Out"=w363:string)  [unwired: 14 in]
            "Magnet Status 2" <- w359
          }
          frame "UI: Level Colors" {
            # "Do not put any code in this frame.\n(It is a separator no-op. You can make a copy of this frame to create a new UI frame)"
            n142 = control-ref of="He LVL Chart"() -> (w366:refnum<vi>)
            n143 = call "Level Color.vi"("LVL Chart Refernce"=w366) -> ()  [unwired: 11 in]
            n144 = control-ref of="N2 LVL Chart"() -> (w365:refnum<vi>)
            n145 = call "Level Color.vi"("LVL Chart Refernce"=w365) -> ()  [unwired: 11 in]
            n146 = call <vilib>:"Add State(s) to Queue__jki_lib_state_machine.vi"("State(s) in (\"\")"=w371) -> ("States Out"=w370:string)  [unwired: 14 in]
          }
          frame "UI: Cursor Set" {
            # "Argument"
            # "Initialize the User Interface, here.\n(this is called automatically, by the Macro: Init)"
            n147 = disable-structure shown="Default" {
              disable-tunnel: w374 -> [w379 w382]
              disable-tunnel: [w379 w381] -> w373
              disable-tunnel: w372 -> [_ w380]
              frame condition #0 {
              }
              frame condition #1 (active) {
                n148 = case shown="\"Idle\", Default" w380 {
                  tunnel: w382 -> [w384 w386]
                  tunnel: [w383 w385] -> w381
                  frame "Idle", Default {
                    n149 = call <vilib>:"Unset Busy.vi"("error in (no error)"=w384) -> ("error out"=w383:errorcluster)  [unwired: 10 in]
                  }
                  frame "Busy" {
                    n150 = call <vilib>:"Set Busy.vi"("error in (no error)"=w386) -> ("error out"=w385:errorcluster)  [unwired: 9 in, 1 out]
                  }
                }
              }
            }
            n151 = call <vilib>:"Add State(s) to Queue__jki_lib_state_machine.vi"("State(s) in (\"\")"=w378) -> ("States Out"=w377:string)  [unwired: 14 in]
          }
          frame "UI: Front Panel State" {
            # "Argument"
            # "Set Front Panel Open or Closed\n(Usage: \"UI: Front Panel State >> Open|Close\")"
            n152 = Unbundle By Name(w390) -> ("Core.Current VI Reference"=w389:refnum<vi>)
            n153 = disable-structure shown="Default" {
              disable-tunnel: w392 -> [w398 w421]
              disable-tunnel: [w397 w421] -> w391
              disable-tunnel: w389 -> [w396 _]
              disable-tunnel: w388 -> [w395 _]
              frame condition #0 (active) {
                n154 = case shown="\"Close\"" w395 {
                  tunnel: w398 -> [w402 w415]
                  tunnel: [w404 w416] -> w397
                  tunnel: w396 -> [w403 w413]
                  frame "Open", Default {
                    n155 = property class="VI"(reference=w403, error in=w402) -> (reference out=w400:refnum<vi>, error out=w401:errorcluster, "FP.State"=w399:T6)
                    n156 = case shown="\"Closed\"" w399 {
                      tunnel: [w407 w410] -> w404
                      tunnel: w401 -> [w406 w410]
                      tunnel: w400 -> [w405 _]
                      frame "Closed" {
                        n157 = invoke class="VI" method="FP.Open"(reference=w405, error in=w406, "Activate"=TRUE, "State"=T6."Standard") -> (error out=w407:errorcluster)  [unwired: 1 in, 4 out]
                      }
                      frame Default {
                      }
                    }
                  }
                  frame "Close" {
                    n158 = property class="VI"(reference=w413, error in=w415) -> (reference out=w412:refnum<vi>, error out=w414:errorcluster, "FP.State"=w411:T6)
                    n159 = case shown="Default" w411 {
                      tunnel: [w417 w420] -> w416
                      tunnel: w414 -> [w417 w419]
                      tunnel: w412 -> [_ w418]
                      frame "Invalid", "Closed" {
                      }
                      frame Default {
                        n160 = invoke class="VI" method="FP.Close"(reference=w418, error in=w419) -> (error out=w420:errorcluster)  [unwired: 1 in, 2 out]
                      }
                    }
                  }
                }
              }
              frame condition #1 {
              }
            }
            n161 = call <vilib>:"Add State(s) to Queue__jki_lib_state_machine.vi"("State(s) in (\"\")"=w394) -> ("States Out"=w393:string)  [unwired: 14 in]
          }
          frame "UI: Minimize" {
            # "Do not put any code in this frame.\n(It is a separator no-op. You can make a copy of this frame to create a new UI frame)"
            n162 = Unbundle By Name(w427) -> ("Core.Current VI Reference"=w426:refnum<vi>)
            n163 = property class="VI"(reference=w426, error in=w423) -> (reference out=w425:refnum<vi>, error out=w424:errorcluster, "Front Panel.PanelBounds"=w431:T12)
            n164 = case shown="\"Min\", Default" w429 {
              tunnel: w431 -> [w434 w442]
              tunnel: [w441 w449] -> w430
              frame "Min", Default {
                n165 = Unbundle By Name(w434) -> ("Left"=w440:i16, "Top"=w438:i16)
                n166 = Add(x=i16 776 ("x 6"), y=w440) -> (x+y=w439:i16)
                n167 = Add(x=w438, y=i16 184 ("x 5")) -> (x+y=w437:i16)
                n168 = Bundle By Name(cluster=w434, "Right"=w439, "Bottom"=w437) -> (w441:T12)
              }
              frame "Max" {
                n169 = Unbundle By Name(w442) -> ("Left"=w448:i16, "Top"=w446:i16)
                n170 = Add(x=i16 1168 ("x 8"), y=w448) -> (x+y=w447:i16)
                n171 = Add(x=w446, y=i16 584 ("x 7")) -> (x+y=w445:i16)
                n172 = Bundle By Name(cluster=w442, "Right"=w447, "Bottom"=w445) -> (w449:T12)
              }
            }
            n173 = property class="VI"(reference=w425, error in=w424, "Front Panel.PanelBounds"=w430) -> (error out=w422:errorcluster)  [unwired: 1 out]
            n174 = call <vilib>:"Add State(s) to Queue__jki_lib_state_machine.vi"("State(s) in (\"\")"=w428) -> ("States Out"=w433:string)  [unwired: 14 in]
          }
          frame "---------- Macro ----------" {
            # "Do not put any code in this frame.\n(It is a separator no-op. You can make a copy of this frame to create a new Macro frame)"
            n175 = call <vilib>:"Add State(s) to Queue__jki_lib_state_machine.vi"("State(s) in (\"\")"=w454) -> ("States Out"=w453:string)  [unwired: 14 in]
          }
          frame "Macro: Initialize" {
            w457 = "UI: Initialize\nUI: Front Panel State >> Open\nUI: Status 2 >> ..."  # UI: Initialize UI: Front Panel State >> Open UI: Status 2 >> ...
            # "Initialization Macro\n(This is called once, when the VI starts)"
            n176 = call <vilib>:"Add State(s) to Queue__jki_lib_state_machine.vi"("State(s) in Front (\"\")"="Data: Initialize\nInitialize Core Data\nEvents: Register", "State(s) in (\"\")"="Process: Sync", "State(s) at Back (\"\")"=w457) -> ("States Out"=w456:string)  [unwired: 12 in]
            n177 = call <vilib>:"Add State(s) to Queue__jki_lib_state_machine.vi"("State(s) in Front (\"\")"=w456, "State(s) in (\"\")"=w463) -> ("States Out"=w462:string)  [unwired: 13 in]
          }
          frame "Macro: Exit" {
            # "Exit Macro\n(This is called once, when the VI exits)"
            n178 = Unbundle By Name(w468) -> ("Core.Close Panel on Exit?"=w474:bool)
            n179 = Select(t="UI: Front Panel State >> Close", s=w474, f="") -> (s? t:f=w471:string)
            n180 = call <vilib>:"Add State(s) to Queue__jki_lib_state_machine.vi"("State(s) in Front (\"\")"="Data: Cleanup\nEvents: Unregister\nProcess: Self Terminate", "State(s) in (\"\")"="Process: Sync", "State(s) at Back (\"\")"="Exit") -> ("States Out"=w465:string)  [unwired: 12 in]
            n181 = call <vilib>:"Add State(s) to Queue__jki_lib_state_machine.vi"("State(s) in (\"\")"=w471, "State(s) at Back (\"\")"=w465) -> ("States Out"=w470:string)  [unwired: 13 in]
            n182 = call <vilib>:"Add State(s) to Queue__jki_lib_state_machine.vi"("State(s) in Front (\"\")"=w470, "State(s) in (\"\")"=w477) -> ("States Out"=w476:string)  [unwired: 13 in]
          }
          frame "---------- Process ----------" {
            # "Template Separator\n(You can make a copy of, or modify, this frame)"
            n183 = call <vilib>:"Add State(s) to Queue__jki_lib_state_machine.vi"("State(s) in (\"\")"=w482) -> ("States Out"=w481:string)  [unwired: 14 in]
          }
          frame "Process: Sync" {
            n184 = Unbundle By Name(w490) -> ("Instrument UI out"=w486:refnum<class "Instrument.OxfordVRM UI.lvclass">)
            n185 = call <vilib>:"WaitOnProcessSync.vi"("error in (no error)"=w485, "SMO"=w486) -> ("error out"=w484:errorcluster, "Don't run?"=w489:bool)  [unwired: 7 in, 1 out]
            n186 = Select(t="Data: Cleanup\nEvents: Unregister\nExit", s=w489, f="") -> (s? t:f=w483:string)
            n187 = call <vilib>:"Add State(s) to Queue__jki_lib_state_machine.vi"("State(s) in Front (\"\")"=w483, "State(s) in (\"\")"=w493) -> ("States Out"=w492:string)  [unwired: 13 in]
          }
          frame "Process: Self Terminate" {
            n188 = Unbundle By Name(w495) -> ("Instrument UI out"=w494:refnum<class "Instrument.OxfordVRM UI.lvclass">)
            n189 = call <vilib>:"SelfTerminate.vi"("error in (no error)"=w497, "SMO in"=w494) -> ("error out"=w496:errorcluster)  [unwired: 8 in, 1 out]
            n190 = call <vilib>:"Add State(s) to Queue__jki_lib_state_machine.vi"("State(s) in (\"\")"=w500) -> ("States Out"=w499:string)  [unwired: 14 in]
          }
          frame "---------- Events ----------" {
            # "Template Separator\n(You can make a copy of, or modify, this frame)"
            n191 = call <vilib>:"Add State(s) to Queue__jki_lib_state_machine.vi"("State(s) in (\"\")"=w505) -> ("States Out"=w504:string)  [unwired: 14 in]
          }
          frame "Events: Register" {
            # "Expand to add\nmore events"
            # "Base Class Protected Events"
            n192 = Unbundle By Name(w519) -> ("Instrument UI out"=w513:refnum<class "Instrument.OxfordVRM UI.lvclass">, "Instrument"=w511:refnum<class "Instrument.OxfordVRM.lvclass">)
            n193 = call <vilib>:"GetProtectedEvents.vi"("SMO"=w513) -> ("error out"=w514:errorcluster, "SMO Protected Events"=w517:T13)  [unwired: 8 in, 1 out]
            n194 = call <userlib>:"Instrument.GetPublicEvents.vi"("Instrument"=w511) -> ("error out"=w512:errorcluster, "Instrument Public Events"=w509:T14, "Instrument out"=w508:refnum<class "Instrument.OxfordVRM.lvclass">)  [unwired: 8 in]
            n195 = call "Instrument.Oxford1820.GetPublicEvents.vi"("Instrument.Oxford1820 in"=w508) -> ("error out"=w506:errorcluster, "OI1820 Public Events"=w507:T15)  [unwired: 8 in, 1 out]
            n196 = register-events(w517, w509, w507) -> (reference out=w518:refnum<event-registration>, error out=w516:errorcluster)  [unwired: 2 in]
            n197 = Merge Errors(w506, w512, w510, w516, w514) -> (w515:errorcluster)
            n198 = call <vilib>:"Add State(s) to Queue__jki_lib_state_machine.vi"("State(s) in (\"\")"=w521) -> ("States Out"=w520:string)  [unwired: 14 in]
          }
          frame "Events: Unregister" {
            n199 = Unregister For Events(event registration refnum=w524, error in=w523) -> (error out=w522:errorcluster)
            n200 = call <vilib>:"Add State(s) to Queue__jki_lib_state_machine.vi"("State(s) in (\"\")"=w527) -> ("States Out"=w526:string)  [unwired: 14 in]
          }
          frame "---------- Action ----------" {
            n201 = Unbundle By Name(w530) -> ("Instrument UI out"=w528:refnum<class "Instrument.OxfordVRM UI.lvclass">)
            n202 = Bundle By Name(cluster=w530, "Instrument UI out"=w528) -> (w529:T9)
            n203 = call <vilib>:"Add State(s) to Queue__jki_lib_state_machine.vi"("State(s) in (\"\")"=w534) -> ("States Out"=w533:string)  [unwired: 14 in]
          }
          frame "Action: Notify UI Closed" {
            # "Notify that the UI has been closed"
            n204 = Unbundle By Name(w537) -> ("Instrument UI out"=w538:refnum<class "Instrument.OxfordVRM UI.lvclass">)
            n205 = call <vilib>:"Hide.vi"("error in (no error)"=w536, "SMO.UI"=w538) -> ("error out"=w535:errorcluster)  [unwired: 8 in, 1 out]
            n206 = call <vilib>:"Add State(s) to Queue__jki_lib_state_machine.vi"("State(s) in (\"\")"=w541) -> ("States Out"=w540:string)  [unwired: 14 in]
          }
          frame "Action: get All" {
            n207 = Unbundle By Name(w542) -> ("Instrument"=w547:refnum<class "Instrument.OxfordVRM.lvclass">)
            n208 = call <userlib>:"Get ALL.vi"("error in (no error)"=w546, "Instrument in"=w547) -> ("error out"=w545:errorcluster, "getAll"=w543:variant, "Instrument out"=w544:refnum<class "Instrument.OxfordVRM.lvclass">)  [unwired: 7 in]
            n209 = Bundle By Name(cluster=w542, "Instrument"=w544, "getAll"=w543) -> (w548:T9)
            n210 = call <vilib>:"Add State(s) to Queue__jki_lib_state_machine.vi"("State(s) in (\"\")"=w551) -> ("States Out"=w550:string)  [unwired: 14 in]
          }
          frame "Action: Hold" {
            n211 = Unbundle By Name(w557) -> ("Instrument"=w555:refnum<class "Instrument.OxfordVRM.lvclass">)
            n212 = call "Instrument.Oxford1820.AbortSequence.vi"("error in (no error)"=w553, "Instrument.Oxford1820"=w555) -> ("error out"=w552:errorcluster, "Instrument.Oxford1820 out"=w554:refnum<class "Instrument.OxfordVRM.lvclass">)  [unwired: 8 in]
            n213 = call "Hold.vi"("error in (no error)"=w552, "Instrument.1820 in"=w554) -> ("error out"=w556:errorcluster)  [unwired: 7 in, 2 out]
            n214 = call <vilib>:"Add State(s) to Queue__jki_lib_state_machine.vi"("State(s) in (\"\")"=w560) -> ("States Out"=w559:string)  [unwired: 14 in]
          }
          frame "Action: To Zero" {
            n215 = Unbundle By Name(w564) -> ("Instrument"=w563:refnum<class "Instrument.OxfordVRM.lvclass">)
            n216 = call "Ramp to Zero.vi"("error in (no error)"=w562, "Instrument.1820 in"=w563) -> ("error out"=w561:errorcluster)  [unwired: 7 in, 2 out]
            n217 = call <vilib>:"Add State(s) to Queue__jki_lib_state_machine.vi"("State(s) in (\"\")"=w567) -> ("States Out"=w566:string)  [unwired: 14 in]
          }
          frame "Action: To Set" {
            n218 = Unbundle By Name(w571) -> ("Instrument"=w570:refnum<class "Instrument.OxfordVRM.lvclass">)
            n219 = call "Ramp to Set.vi"("error in (no error)"=w569, "Instrument.1820 in"=w570) -> ("error out"=w568:errorcluster)  [unwired: 7 in, 2 out]
            n220 = call <vilib>:"Add State(s) to Queue__jki_lib_state_machine.vi"("State(s) in (\"\")"=w574) -> ("States Out"=w573:string)  [unwired: 14 in]
          }
          frame "Action: Clamp" {
            n221 = Unbundle By Name(w575) -> ("Instrument"=w578:refnum<class "Instrument.OxfordVRM.lvclass">)
            n222 = call "Clamp.vi"("error in (no error)"=w577, "Instrument.1820 in"=w578) -> ("error out"=w576:errorcluster)  [unwired: 7 in, 2 out]
            n223 = call <vilib>:"Add State(s) to Queue__jki_lib_state_machine.vi"("State(s) in (\"\")"=w581) -> ("States Out"=w580:string)  [unwired: 14 in]
          }
          frame "Action: Fill" {
            n224 = Unbundle By Name(w589) -> ("Instrument"=w588:refnum<class "Instrument.OxfordVRM.lvclass">)
            n225 = Select(t=T7 "OFF" ("Fill Mode"), s="Fast/Slow Fill", f=T7 "ON" ("Fill Mode")) -> (s? t:f=w584:T7)
            n226 = call "Set Fill Mode.vi"("error in (no error)"=w587, "Fill Mode"=w584, "Instrument.1820 in"=w588) -> ("error out"=w586:errorcluster)  [unwired: 6 in, 2 out]
            n227 = call <vilib>:"Add State(s) to Queue__jki_lib_state_machine.vi"("State(s) in (\"\")"=w592) -> ("States Out"=w591:string)  [unwired: 14 in]
          }
          frame "Action: LPF" {
            n228 = Unbundle By Name(w595) -> ("Instrument"=w602:refnum<class "Instrument.OxfordVRM.lvclass">)
            n229 = Select(t=T3 "ON" ("LPF State"), s="LPF Power", f=T3 "OFF" ("LPF State")) -> (s? t:f=w599:T3)
            n230 = call "Set LPF State.vi"("error in (no error)"=w601, "LPF State"=w599, "Instrument.1820 in"=w602) -> ("error out"=w600:errorcluster)  [unwired: 6 in, 2 out]
            n231 = Get Date/Time In Seconds() -> (seconds since 1Jan1904=w593:timestamp)
            n232 = Bundle By Name(cluster=w595, "LPF time"=w593) -> (w594:T9)
            n233 = call <vilib>:"Add State(s) to Queue__jki_lib_state_machine.vi"("State(s) in (\"\")"=w605) -> ("States Out"=w604:string)  [unwired: 14 in]
          }
          frame "Action: Needle Valve" {
            # "2=open"
            # "1=closed"
            n234 = Unbundle By Name(w615) -> ("Instrument"=w614:refnum<class "Instrument.OxfordVRM.lvclass">)
            n235 = Build Array("Close Needle Valve", "Open Needle Valve") -> (w612:bool[])
            n236 = Boolean Array To Number(Boolean array=w612) -> (number=w609:u32)
            n237 = case shown="1, Default" w609 {
              tunnel: [0.0 ("Needle Valve (%)") "Open Target"] -> w608
              frame 1, Default {
              }
              frame 2 {
              }
            }
            n238 = call "Set Needle Valve.vi"("error in (no error)"=w613, "Needle Valve (%)"=w608, "Instrument.1820 in"=w614) -> ("error out"=w607:errorcluster)  [unwired: 6 in, 2 out]
            n239 = flat-sequence {
              tunnel: [w619] -> w606
              tunnel: w607 -> [w619]
              frame #0 {
                n240 = local write "Close Needle Valve"(FALSE ("Close Needle Valve")) -> ()
                n241 = local write "Open Needle Valve"(FALSE ("Open Needle Valve")) -> ()
              }
            }
            n242 = call <vilib>:"Add State(s) to Queue__jki_lib_state_machine.vi"("State(s) in (\"\")"=w618) -> ("States Out"=w617:string)  [unwired: 14 in]
          }
          frame "Action: PS Heat" {
            n243 = Unbundle By Name(w628) -> ("Instrument"=w625:refnum<class "Instrument.OxfordVRM.lvclass">)
            n244 = call "Set Switch Heater.vi"("error in (no error)"=w630, "Switch Heater"=w624, "Instrument.1820 in"=w625) -> ("error out"=w629:errorcluster)  [unwired: 6 in, 2 out]
            n245 = Get Date/Time In Seconds() -> (seconds since 1Jan1904=w627:timestamp)
            n246 = Bundle By Name(cluster=w628, "switch time"=w627) -> (w626:T9)
            n247 = call <vilib>:"Add State(s) to Queue__jki_lib_state_machine.vi"("State(s) in (\"\")"=w633) -> ("States Out"=w632:string)  [unwired: 14 in]
          }
          frame "Action: Send to IPS" {
            n248 = Unbundle By Name(w639) -> ("Instrument"=w638:refnum<class "Instrument.OxfordVRM.lvclass">)
            n249 = call "Set Target.vi"("error in (no error)"=w637, "Target Rate (T/min)"="Target Rate (T/min)", "Target Field (T)"="Target Field (T)", "Instrument.1820 in"=w638) -> ("error out"=w636:errorcluster)  [unwired: 5 in, 2 out]
            n250 = call <vilib>:"Add State(s) to Queue__jki_lib_state_machine.vi"("State(s) in (\"\")"=w642) -> ("States Out"=w641:string)  [unwired: 14 in]
          }
        }
      }
    }
    frame Error {
    }
  }
  n251 = call-parent "Process.vi"("error in"=w9, "Instrument UI in"=w8) -> ("error out"=w6:errorcluster, "Instrument UI out"=→"Oxford1820 UI out":refnum<class "Instrument.OxfordVRM UI.lvclass">)  [unwired: 8 in]
  n252 = disable-structure shown="Disabled" {
    frame Disabled {
    }
    frame Enabled {
    }
  }
  n253 = Merge Errors(w6, w5) -> (→"error out":errorcluster)
  "version" <- "v20/12/08" ("version")
